vi "Process Node.vi"(8 "error in (no error)":errorcluster, 9 "inspect dependencies":bool, 10 "level":i32, 11 "node ref":refnum<vi>) -> (0 "error out":errorcluster)   [LabVIEW 2014, in "lvprj2html.lvlib"]
uses:
  lvprj2html.lvlib
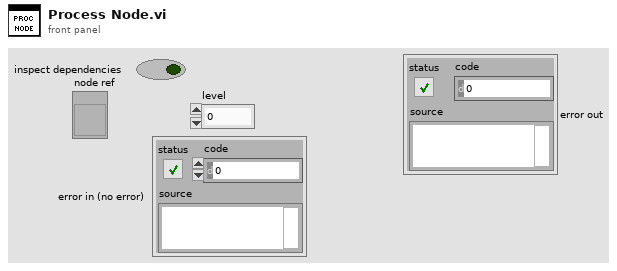
[diagram p1: front panel]
types:
  T1 = typedef "LVRectTypeDef.ctl" = cluster{"Left":i16, "Top":i16, "Right":i16, "Bottom":i16}
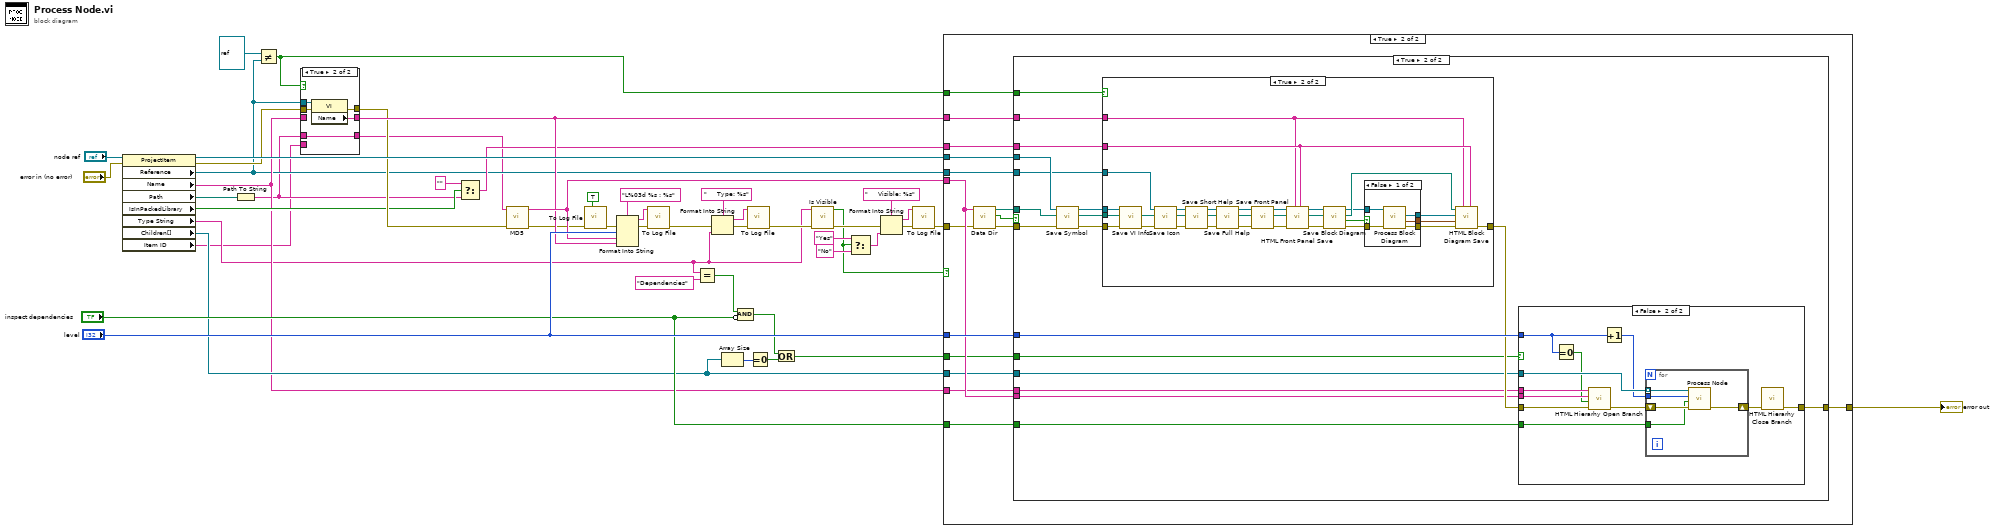
[diagram p0: block diagram]
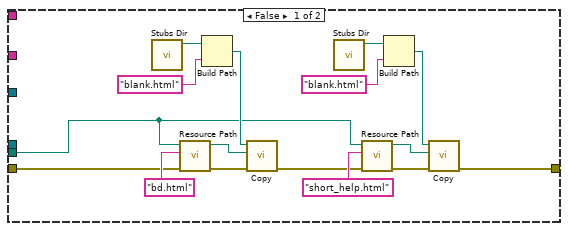
[diagram p4: hidden frame]
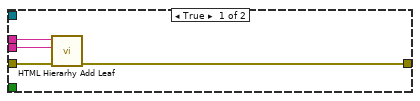
[diagram p6: hidden frame]
diagram:
  n1 = property class="ProjectItem"(reference="node ref", error in="error in (no error)") -> (reference out=w45:refnum<vi>, error out=w37:errorcluster, "Reference"=w4:refnum<vi>, "Name"=w15:string, "Path"=w18:path, "IsInPackedLibrary"=w19:bool, "Type String"=w5:string, "Children[]"=w21:refnum<vi>[], "Item ID"=w2:string)
  n2 = Path To String(path=w18) -> (string=w3:string)
  n3 = Not Equal?(x=refnum<vi> refnum ("reference out"), y=w4) -> (x != y?=w39:bool)
  n4 = case shown="True" w39 {
    tunnel: [w52 w57] -> w38
    tunnel: w4 -> [_ w56]
    tunnel: w15 -> [w52 _]
    tunnel: w37 -> [w51 w55]
    tunnel: [w51 w54] -> w20
    tunnel: w3 -> [_ w53]
    tunnel: w2 -> [w50 _]
    tunnel: [w50 w53] -> w1
    frame False {
    }
    frame True {
      n5 = property class="VI"(reference=w56, error in=w55) -> (error out=w54:errorcluster, "Name"=w57:string)  [unwired: 1 out]
    }
  }
  n6 = Select(t="" ("f"), s=w19, f=w3) -> (s? t:f=w36:string)
  n7 = call "MD5.vi"("error in (no error)"=w20, "Input String"=w1) -> ("error out"=w23:errorcluster, "MD5 message-digest"=w41:string)  [unwired: 8 in]
  n8 = call "To Log File.vi"("new line"=TRUE, "error in (no error)"=w23) -> ("error out"=w24:errorcluster)  [unwired: 9 in]
  n9 = Format Into String(format string="L%03d %s : %s", error in=w24, "level", w41, w38) -> (resulting string=w48:string, error out=w43:errorcluster)  [unwired: 1 in]
  n10 = call "To Log File.vi"("error in (no error)"=w43, "string"=w48) -> ("error out"=w34:errorcluster)  [unwired: 9 in]
  n11 = Equal?(x=w5, y="Dependencies") -> (x = y?=w29:bool)
  n12 = Format Into String(format string="     Type: %s", error in=w34, w5) -> (resulting string=w32:string, error out=w33:errorcluster)  [unwired: 1 in]
  n13 = Array Size(array=w21) -> (size(s)=w30:i32)
  n14 = Compound Arithmetic op=AND(w29, invert "inspect dependencies") -> (w27:bool)
  n15 = call "To Log File.vi"("error in (no error)"=w33, "string"=w32) -> ("error out"=w16:errorcluster)  [unwired: 9 in]
  n16 = Equal To 0?(x=w30) -> (x = 0?=w28:bool)
  n17 = Compound Arithmetic op=OR(w27, w28) -> (w26:bool)
  n18 = call "Is Visible.vi"("error in"=w16, "type str"=w5) -> ("error out"=w12:errorcluster, "yes"=w6:bool)  [unwired: 8 in]
  n19 = Select(t="Yes" ("y"), s=w6, f="No" ("y")) -> (s? t:f=w9:string)
  n20 = Format Into String(format string="     Visible: %s", error in=w12, w9) -> (resulting string=w10:string, error out=w13:errorcluster)  [unwired: 1 in]
  n21 = call "To Log File.vi"("error in (no error)"=w13, "string"=w10) -> ("error out"=w14:errorcluster)  [unwired: 9 in]
  n22 = case shown="True" w6 {
    tunnel: "level" -> [_ w74]
    tunnel: w45 -> [_ w73]
    tunnel: [w58 w70] -> w42
    tunnel: w41 -> [_ w69]
    tunnel: w4 -> [_ w68]
    tunnel: w15 -> [_ w67]
    tunnel: w39 -> [_ w65]
    tunnel: w38 -> [_ w64]
    tunnel: w36 -> [_ w63]
    tunnel: w14 -> [w58 w62]
    tunnel: w26 -> [_ w61]
    tunnel: "inspect dependencies" -> [_ w60]
    tunnel: w21 -> [_ w59]
    frame False {
    }
    frame True {
      n23 = call "Data Dir.vi"("error in (no error)"=w62, "Name"=w69) -> ("error out"=w71:errorcluster, "created"=w66:bool, "path"=w72:path)  [unwired: 7 in]
      n24 = case shown="True" w66 {
        tunnel: w74 -> [_ w93]
        tunnel: w73 -> [_ w92]
        tunnel: w72 -> [_ w91]
        tunnel: w71 -> [w75 w87]
        tunnel: w63 -> [_ w86]
        tunnel: [w75 w84] -> w70
        tunnel: w59 -> [_ w83]
        tunnel: w69 -> [_ w82]
        tunnel: w68 -> [_ w81]
        tunnel: w67 -> [_ w80]
        tunnel: w65 -> [_ w79]
        tunnel: w64 -> [_ w78]
        tunnel: w61 -> [_ w77]
        tunnel: w60 -> [_ w76]
        frame False {
        }
        frame True {
          n25 = call "Save Symbol.vi"("error in (no error)"=w87, "path"=w91, "proj ref"=w92) -> ("error out"=w89:errorcluster, "path out"=w88:path, "proj ref out"=w90:refnum<vi>)  [unwired: 6 in]
          n26 = case shown="True" w79 {
            tunnel: w81 -> [_ w131]
            tunnel: w90 -> [_ w140]
            tunnel: w86 -> [_ w119]
            tunnel: w89 -> [w104 w133]
            tunnel: [w95 w120] -> w85
            tunnel: w88 -> [w96 w132]
            tunnel: w78 -> [_ w115]
            frame False {
              n27 = call "Stubs Dir.vi"() -> ("path"=w109:path)  [unwired: 11 in]
              n28 = call "Resource Path.vi"("error in (no error)"=w104, "resource file name"="bd.html", "data dir"=w96) -> ("error out"=w105:errorcluster, "path"=w106:path)  [unwired: 7 in]
              n29 = Build Path(base path=w109, name or relative path="blank.html") -> (appended path=w108:path)
              n30 = call "Copy.vi"("error in (no error)"=w105, "dst"=w106, "src"=w108) -> ("error out"=w97:errorcluster)  [unwired: 8 in]
              n31 = call "Stubs Dir.vi"() -> ("path"=w99:path)  [unwired: 11 in]
              n32 = call "Resource Path.vi"("error in (no error)"=w97, "resource file name"="short_help.html", "data dir"=w96) -> ("error out"=w103:errorcluster, "path"=w102:path)  [unwired: 7 in]
              n33 = Build Path(base path=w99, name or relative path="blank.html") -> (appended path=w100:path)
              n34 = call "Copy.vi"("error in (no error)"=w103, "dst"=w102, "src"=w100) -> ("error out"=w95:errorcluster)  [unwired: 8 in]
            }
            frame True {
              n35 = call "Save VI Info.vi"("error in (no error)"=w133, "path"=w132, "node ref"=w140) -> ("error out"=w130:errorcluster, "path out"=w129:path)  [unwired: 6 in, 1 out]
              n36 = call "Save Icon.vi"("error in (no error)"=w130, "path"=w129, "vi ref"=w131) -> ("error out"=w134:errorcluster, "path out"=w135:path, "reference out"=w136:refnum<vi>)  [unwired: 6 in]
              n37 = call "Save Short Help.vi"("error in (no error)"=w134, "path"=w135, "vi ref"=w136) -> ("error out"=w137:errorcluster, "path out"=w138:path, "reference out"=w139:refnum<vi>)  [unwired: 6 in]
              n38 = call "Save Full Help.vi"("error in (no error)"=w137, "path"=w138, "vi ref"=w139) -> ("error out"=w124:errorcluster, "path out"=w125:path, "reference out"=w126:refnum<vi>)  [unwired: 6 in]
              n39 = call "Save Front Panel.vi"("error in (no error)"=w124, "path"=w125, "vi ref"=w126) -> ("error out"=w123:errorcluster, "path out"=w128:path, "reference out"=w127:refnum<vi>)  [unwired: 6 in]
              n40 = call "HTML Front Panel Save.vi"("url"=w119, "title"=w115, "error in"=w123, "path"=w128, "vi ref"=w127) -> ("error out"=w111:errorcluster, "path out"=w122:path, "vi ref out"=w110:refnum<vi>)  [unwired: 4 in]
              n41 = call "Save Block Diagram.vi"("error in (no error)"=w111, "path"=w122, "vi ref"=w110) -> ("error out"=w112:errorcluster, "unavailable"=w114:bool, "path out"=w118:path, "reference out"=w113:refnum<vi>)  [unwired: 5 in]
              n42 = case shown="False" w114 {
                tunnel: w113 -> [w145 _]
                tunnel: w112 -> [w144 w146]
                tunnel: [w143 w146] -> w121
                tunnel: [w142 _] -> w117
                tunnel: [w141 _] -> w116
                frame False {
                  n43 = call "Process Block Diagram.vi"("error in (no error)"=w144, "vi ref"=w145) -> ("error out"=w143:errorcluster, "sub vi loc"=w141:T1[], "sub vi refs"=w142:refnum<vi>[])  [unwired: 7 in]
                }
                frame True {
                }
              }
              n44 = call "HTML Block Diagram Save.vi"("url"=w119, "title"=w115, "error in"=w121, "sub vi loc"=w116, "sub vi refs"=w117, "base path"=w118) -> ("error out"=w120:errorcluster)  [unwired: 5 in]
            }
          }
          n45 = case shown="False" w77 {
            tunnel: w83 -> [_ w161]
            tunnel: w80 -> [w150 w160]
            tunnel: w82 -> [w149 w159]
            tunnel: w93 -> [_ w158]
            tunnel: w85 -> [w147 w153]
            tunnel: [w148 w152] -> w84
            tunnel: w76 -> [_ w151]
            frame True {
              n46 = call "HTML Hierarhy Add Leaf.vi"("error in"=w147, "id"=w149, "label"=w150) -> ("error out"=w148:errorcluster)  [unwired: 8 in]
            }
            frame False {
              n47 = Equal To 0?(x=w158) -> (x = 0?=w155:bool)
              n48 = call "HTML Hierarhy Open Branch.vi"("error in"=w153, "checked"=w155, "id"=w159, "label"=w160) -> ("error out"=w156:errorcluster)  [unwired: 7 in]
              n49 = Increment(x=w158) -> (x+1=w154:i32)
              n50 = for {
                tunnel: w161 -> [w166] mode=indexing
                tunnel: w154 -> [w165]
                shift-right: [w164] -> w157
                shift-left: w156 -> [w163]
                tunnel: w151 -> [w162]
                n51 = call "Process Node.vi"("error in (no error)"=w163, "inspect dependencies"=w162, "level"=w165, "node ref"=w166) -> ("error out"=w164:errorcluster)  [unwired: 7 in]
              }
              n52 = call "HTML Hierarhy Close Branch.vi"("error in"=w157) -> ("error out"=w152:errorcluster)  [unwired: 10 in]
            }
          }
        }
      }
    }
  }
  "error out" <- w42
